vi "Create RxTx.vi"(8 "error in (no error)":errorcluster, 11 "Channel in":refnum<class "Channel.lvclass">) -> (0 "error out":errorcluster, 3 "Channel out":refnum<class "Channel.lvclass">)   [LabVIEW 2018, in "Channel.lvclass"]
doc: "Create the queres responsible for communication"
uses:
  Channel.lvclass
  Channel.lvclass/Channel.ctl
  RxTx/CCS_RxTx.lvclass
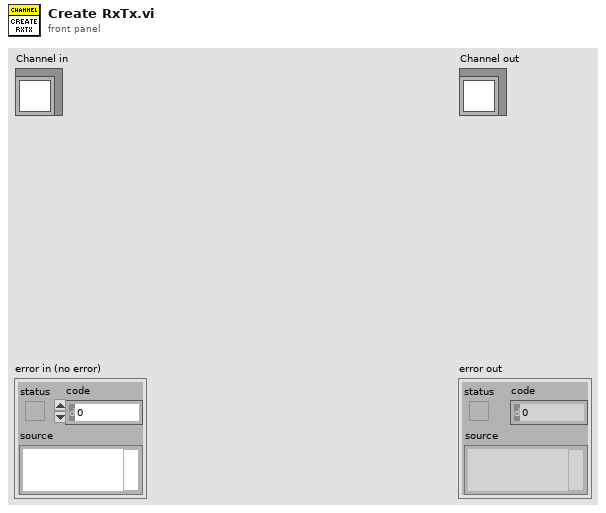
[diagram p1: front panel]
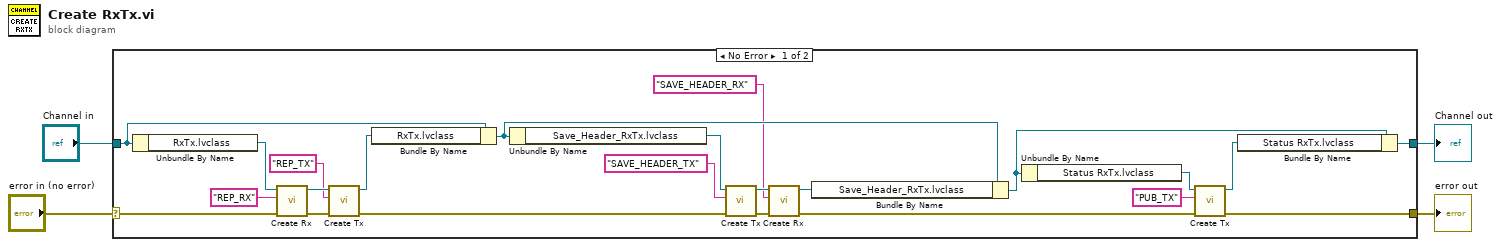
[diagram p0: block diagram]
diagram:
  n1 = case shown="No Error" "error in (no error)" {
    selector: "error in (no error)" -> [w20 w29]
    tunnel: [w7 w29] -> w3
    tunnel: [w6 w28] -> w1
    tunnel: "Channel in" -> [w24 w28]
    frame No Error {
      n2 = Unbundle By Name(w24) -> ("RxTx.lvclass"=w26:refnum<class "CCS_RxTx.lvclass">)
      n3 = call "Create Rx.vi"("error in (no error)"=w20, "Reader Name"="REP_RX", "RxTx in"=w26) -> ("error out"=w27:errorcluster, "RxTx out"=w25:refnum<class "CCS_RxTx.lvclass">)  [unwired: 7 in]
      n4 = call "Create Tx.vi"("error in (no error)"=w27, "Writer Name"="REP_TX", "RxTx in"=w25) -> ("error out"=w13:errorcluster, "RxTx out"=w14:refnum<class "CCS_RxTx.lvclass">)  [unwired: 7 in]
      n5 = Bundle By Name(cluster=w24, "RxTx.lvclass"=w14) -> (w21:refnum<class "Channel.lvclass">)
      n6 = Unbundle By Name(w21) -> ("Save_Header_RxTx.lvclass"=w23:refnum<class "CCS_RxTx.lvclass">)
      n7 = call "Create Tx.vi"("error in (no error)"=w13, "Writer Name"="SAVE_HEADER_TX", "RxTx in"=w23) -> ("error out"=w18:errorcluster, "RxTx out"=w17:refnum<class "CCS_RxTx.lvclass">)  [unwired: 7 in]
      n8 = call "Create Rx.vi"("error in (no error)"=w18, "Reader Name"="SAVE_HEADER_RX", "RxTx in"=w17) -> ("error out"=w9:errorcluster, "RxTx out"=w19:refnum<class "CCS_RxTx.lvclass">)  [unwired: 7 in]
      n9 = Bundle By Name(cluster=w21, "Save_Header_RxTx.lvclass"=w19) -> (w11:refnum<class "Channel.lvclass">)
      n10 = Unbundle By Name(w11) -> ("Status RxTx.lvclass"=w12:refnum<class "CCS_RxTx.lvclass">)
      n11 = call "Create Tx.vi"("error in (no error)"=w9, "Writer Name"="PUB_TX", "RxTx in"=w12) -> ("error out"=w7:errorcluster, "RxTx out"=w10:refnum<class "CCS_RxTx.lvclass">)  [unwired: 7 in]
      n12 = Bundle By Name(cluster=w11, "Status RxTx.lvclass"=w10) -> (w6:refnum<class "Channel.lvclass">)
    }
    frame Error {
    }
  }
  "error out" <- w3
  "Channel out" <- w1
